vi "Camera.vi"() -> ()   [LabVIEW 2015]
uses:
  <vilib>/rvi/Emulation/niFpgaGetClockAttributes.vi
  <vilib>/rvi/Emulation/niFpgaSctlEmulationGetInTimedLoop.vi
  <vilib>/rvi/Emulation/niFpgaEmulationReportErrorSimple.vi
  <vilib>/rvi/eio/common/nirviEmuTemplateMethod_errors.vi
  <vilib>/rvi/Emulation/niFpgaCriticalErrorInLSC.vi
  <vilib>/eio/EIONode/EIONode.xnode
panel:
  out "Camera flash time":i16
  in  "Camera flash":i16
  in  "Camera offset x":i16=98
  in  "Flash":bool
  # "** Trigger the fluorenscence camera (100 - x ) *100 microseconds earlier"
  # "** Camera flash is set to be the time for triggering the flash at the end of every video.\n** The unit is second."
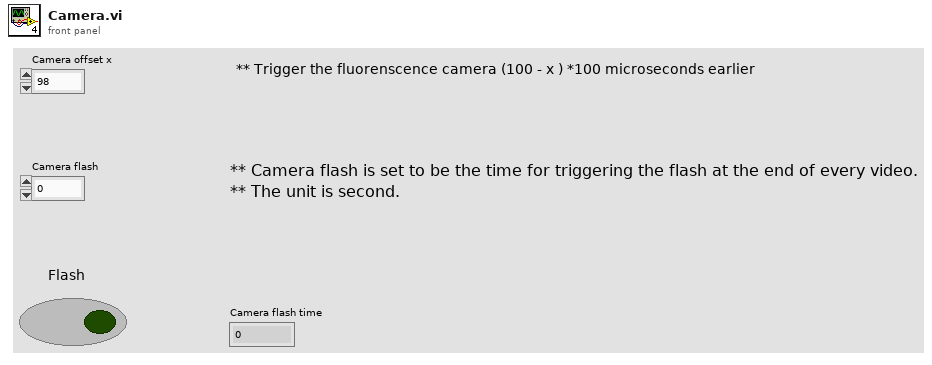
[diagram p1: front panel]
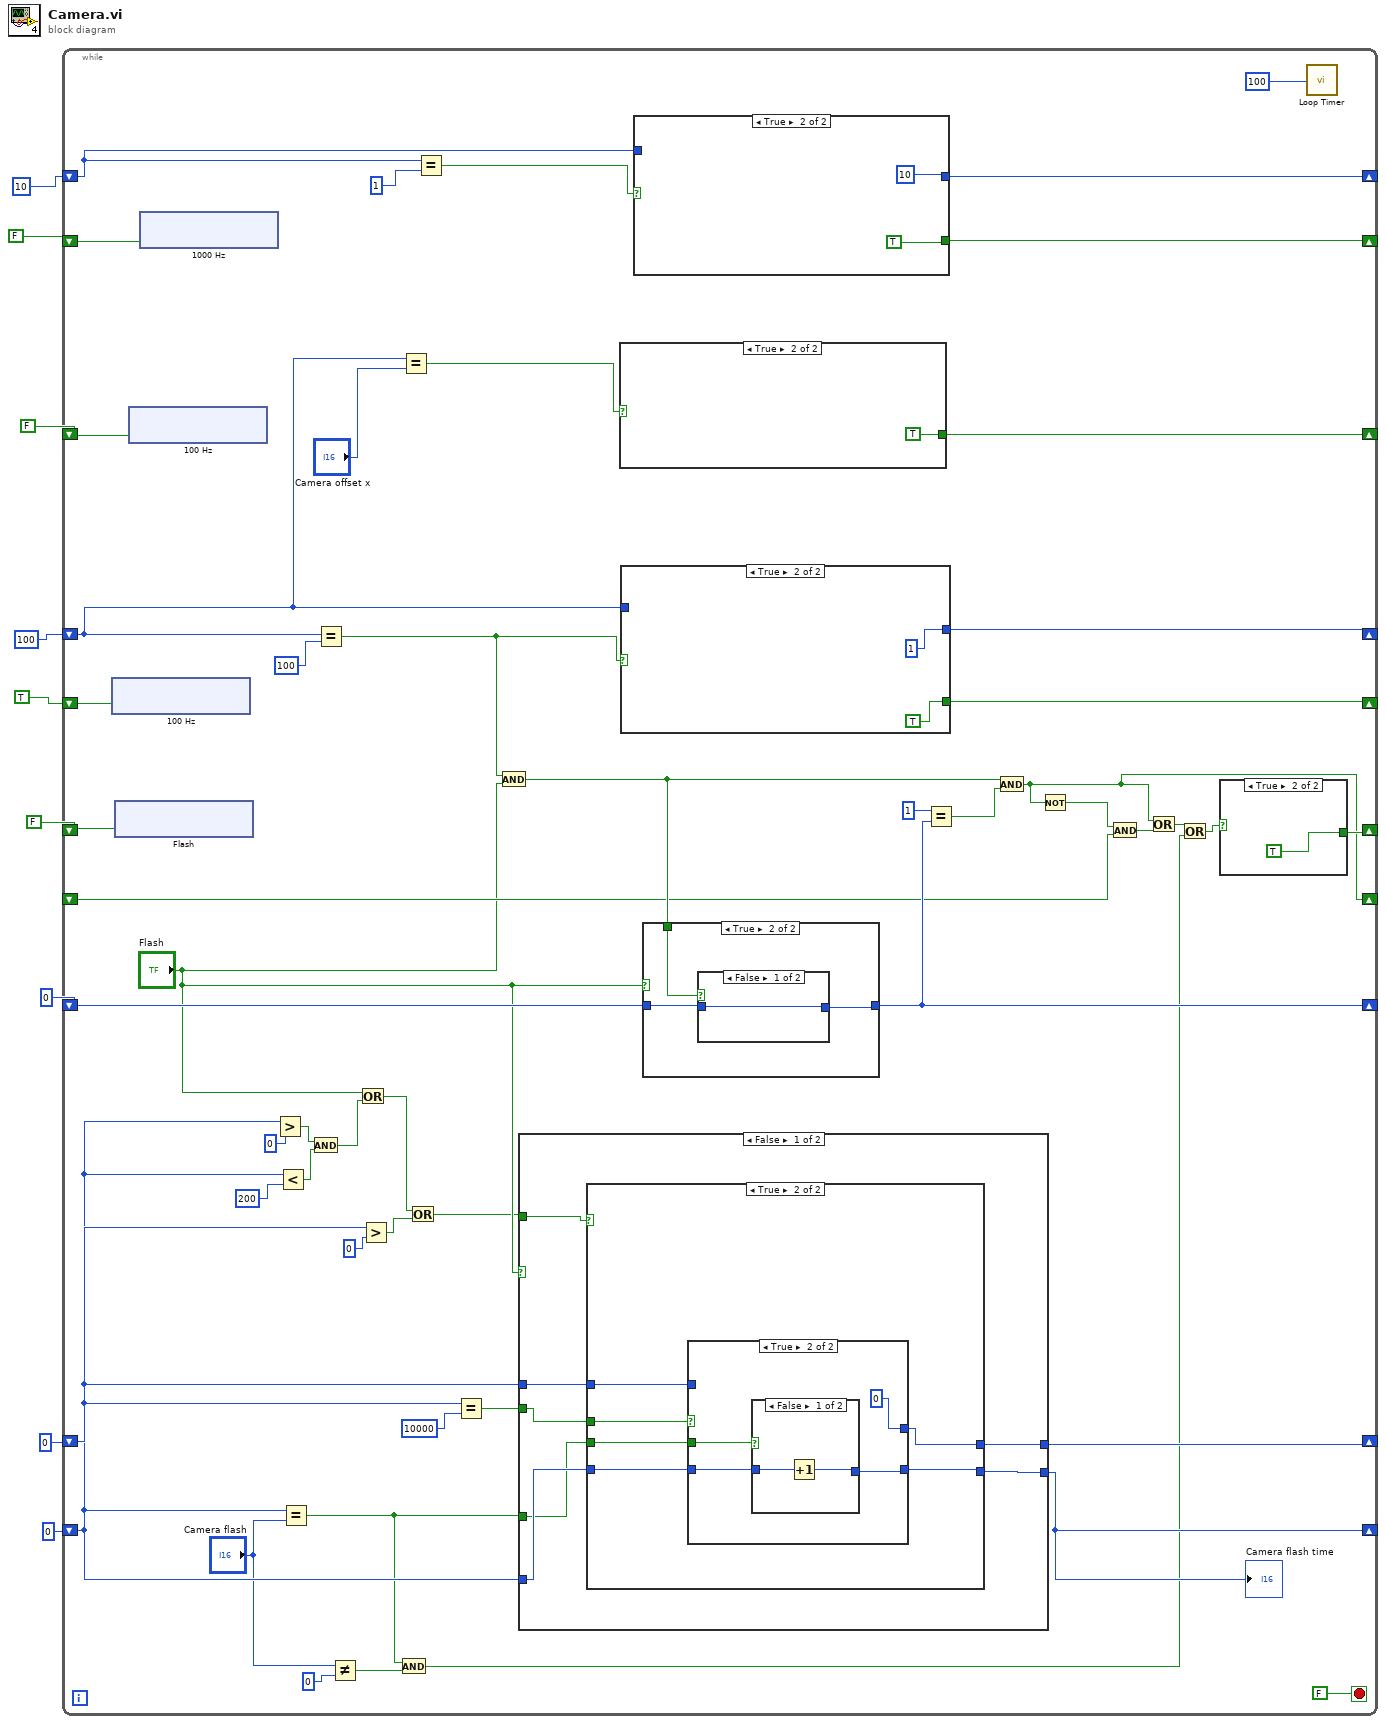
[diagram p0: block diagram]
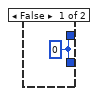
[diagram p2: hidden frame]
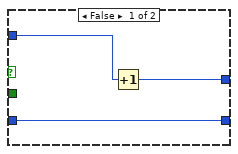
[diagram p3: hidden frame]
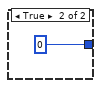
[diagram p4: hidden frame]
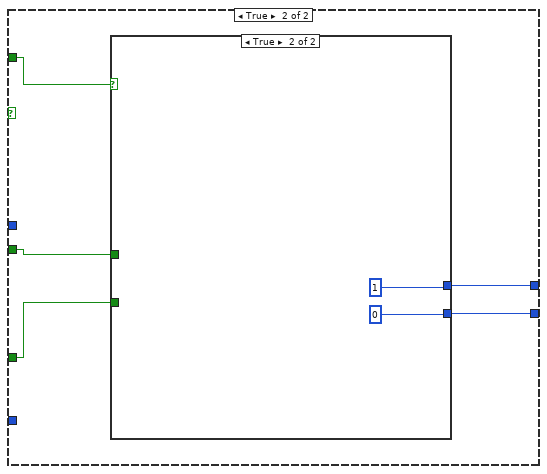
[diagram p5: hidden frame]
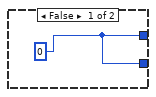
[diagram p6: hidden frame]
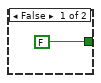
[diagram p7: hidden frame]
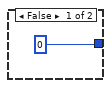
[diagram p8: hidden frame]
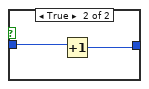
[diagram p9: hidden frame]
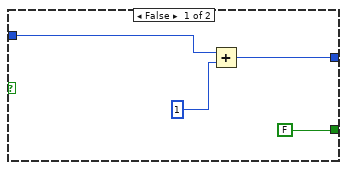
[diagram p10: hidden frame]
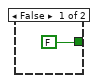
[diagram p11: hidden frame]
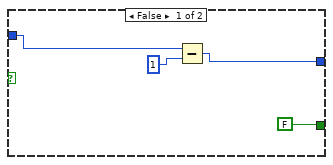
[diagram p12: hidden frame]
diagram:
  n1 = while {
    shift-right: [w60] -> _
    shift-left: FALSE -> [w61]
    shift-right: [w57] -> _
    shift-left: i16 10 -> [w50]
    shift-right: [w54] -> _
    shift-left: FALSE -> [w55]
    shift-right: [w53] -> _
    shift-left: TRUE -> [w46]
    shift-right: [w52] -> _
    shift-left: i16 100 -> [w41]
    shift-right: [w43] -> _
    shift-left: i16 0 -> [w47]
    shift-right: [w39] -> _
    shift-left: FALSE -> [w40]
    shift-right: [w35] -> _
    shift-left: _ -> [w36]
    shift-right: [w28] -> _
    shift-left: i16 0 -> [w21]
    shift-right: [w29] -> _
    shift-left: i16 0 -> [w15]
    stop <- FALSE stop-if-true
    n2 = xnode "100 Hz"("ConnectorC/DIO2"=w46) -> ()  [unwired: 1 in, 1 out]
    n3 = xnode "Flash"("ConnectorC/DIO3"=w40) -> ()  [unwired: 1 in, 1 out]
    n4 = xnode "100 Hz"("ConnectorC/DIO1"=w55) -> ()  [unwired: 1 in, 1 out]
    n5 = xnode "1000 Hz"("ConnectorC/DIO0"=w61) -> ()  [unwired: 1 in, 1 out]
    n6 = Greater?(x=w15, y=i16 0) -> (0:w18:bool)
    n7 = Less?(x=w15, y=i16 200) -> (x < y?=w17:bool)
    n8 = Equal?(x=w15, y="Camera flash") -> (x = y?=w11:bool)
    n9 = And(x=w18, y=w17) -> (x .and. y?=w16:bool)
    n10 = Equal?(x=w41, y=i16 100) -> (x = y?=w48:bool)
    n11 = Not Equal?(x="Camera flash", y=i16 0) -> (x != y?=w12:bool)
    n12 = Or(x="Flash", y=w16) -> (x .or. y?=w23:bool)
    n13 = Greater?(x=w21, y=i16 0) -> (0:w24:bool)
    n14 = And(x=w11, y=w12) -> (x .and. y?=w10:bool)
    n15 = Equal?(x=w41, y="Camera offset x") -> (x = y?=w56:bool)
    n16 = Or(x=w23, y=w24) -> (x .or. y?=w22:bool)
    n17 = Equal?(x=w50, y=i16 1) -> (x = y?=w49:bool)
    n18 = Equal?(x=w21, y=i16 10000) -> (x = y?=w27:bool)
    n19 = And(x=w48, y="Flash") -> (x .and. y?=w45:bool)
    n20 = case shown="False" "Flash" {
      tunnel: [w67 w90] -> w29
      tunnel: [w68 w89] -> w28
      tunnel: w21 -> [w65 _]
      tunnel: w27 -> [w66 w88]
      tunnel: w11 -> [w62 w87]
      tunnel: w15 -> [w64 _]
      tunnel: w22 -> [w63 w86]
      frame False {
        n21 = case shown="True" w63 {
          tunnel: [w69 w73] -> w68
          tunnel: [w69 w72] -> w67
          tunnel: w66 -> [_ w75]
          tunnel: w65 -> [_ w74]
          tunnel: w64 -> [_ w71]
          tunnel: w62 -> [_ w70]
          frame False {
            w69 = i16 0
          }
          frame True {
            n22 = case shown="True" w75 {
              tunnel: w74 -> [w78 _]
              tunnel: [w77 i16 0] -> w73
              tunnel: [w76 w81] -> w72
              tunnel: w71 -> [w76 w80]
              tunnel: w70 -> [_ w79]
              frame False {
                n23 = Increment(x=w78) -> (x+1=w77:i16)
              }
              frame True {
                n24 = case shown="False" w79 {
                  tunnel: [w83 i16 0] -> w81
                  tunnel: w80 -> [w84 _]
                  frame False {
                    n25 = Increment(x=w84) -> (x+1=w83:i16)
                  }
                  frame True {
                  }
                }
              }
            }
          }
        }
      }
      frame True {
        n26 = case shown="True" w86 {
          tunnel: [w91 i16 1] -> w89
          tunnel: w87 -> [_ _]
          tunnel: [w91 i16 0] -> w90
          tunnel: w88 -> [_ _]
          frame False {
            w91 = i16 0
          }
          frame True {
          }
        }
      }
    }
    "Camera flash time" <- w29
    n27 = case shown="True" w56 {
      tunnel: [FALSE TRUE] -> w54
      frame False {
      }
      frame True {
      }
    }
    n28 = case shown="True" w48 {
      tunnel: [FALSE TRUE] -> w53
      tunnel: [w104 i16 1] -> w52
      tunnel: w41 -> [w106 _]
      frame False {
        n29 = Add(x=w106, y=i16 1) -> (x+y=w104:i16)
      }
      frame True {
      }
    }
    n30 = case shown="True" w49 {
      tunnel: [w111 i16 10] -> w57
      tunnel: [FALSE TRUE] -> w60
      tunnel: w50 -> [w112 _]
      frame False {
        n31 = Subtract(x=w112, y=i16 1) -> (x-y=w111:i16)
      }
      frame True {
      }
    }
    n32 = case shown="True" "Flash" {
      tunnel: w47 -> [_ w98]
      tunnel: [i16 0 w97] -> w43
      tunnel: w45 -> [_ w99]
      frame False {
      }
      frame True {
        n33 = case shown="False" w99 {
          tunnel: w98 -> [w100 w102]
          tunnel: [w100 w101] -> w97
          frame False {
          }
          frame True {
            n34 = Increment(x=w102) -> (x+1=w101:i16)
          }
        }
      }
    }
    n35 = Equal?(x=i16 1, y=w43) -> (x = y?=w42:bool)
    n36 = And(x=w45, y=w42) -> (x .and. y?=w35:bool)
    n37 = Not(x=w35) -> (.not. x?=w37:bool)
    n38 = And(x=w37, y=w36) -> (x .and. y?=w38:bool)
    n39 = Or(x=w35, y=w38) -> (x .or. y?=w32:bool)
    n40 = Or(x=w32, y=w10) -> (x .or. y?=w31:bool)
    n41 = case shown="True" w31 {
      tunnel: [FALSE TRUE] -> w39
      frame False {
      }
      frame True {
      }
    }
    n42 = call "Loop Timer"("Count(uSec)"=u32 100) -> ()  [unwired: 1 out]
  }
